vi "Read Caller Actor Name.vi"(11 "Command Message Interface in":refnum<class "Command Message Interface.lvclass">) -> (2 "Caller Actor Name":string, 3 "Command Message Interface out":refnum<class "Command Message Interface.lvclass">)   [LabVIEW 2016, in "Stream Mediator.lvlib" / "Command Message Interface.lvclass"]
doc: "--\nCopyright © 2017 Composed SystemsI All rights reserved.\n\nAuthor: Jon McBee <jon.mcbee@composed.io>\n\nThis library is provided \"AS IS\" ,WITHOUT WARRANTIES OR\nCONDITIONS OF ANY KIND, either express or implied.\n\nComposed Systems -- composed.io\n\nStream 0.0.1.1\nJon McBee - Composed Systems\nCopyright (c) 2017, Composed Systems"
uses:
  <userlib>/Composed Systems/Stream/Mediator/Classes/Message Command Interface/Command Message Interface.lvclass
  <userlib>/Composed Systems/Stream/Mediator/Classes/Message Command Interface/Command Message Interface.lvclass/Command Message Interface.ctl
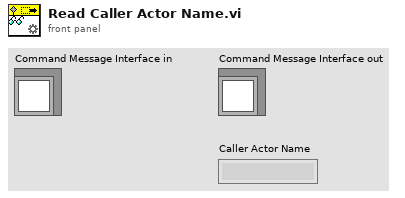
[diagram p1: front panel]
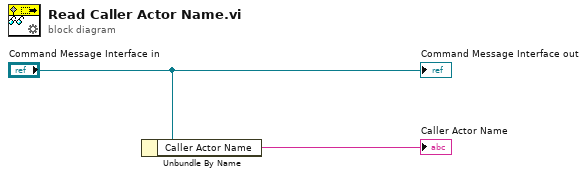
[diagram p0: block diagram]
diagram:
  n1 = Unbundle By Name("Command Message Interface in") -> ("Caller Actor Name"=→"Caller Actor Name":string)
  "Command Message Interface out" <- "Command Message Interface in"
